vi "Setup.vi"(11 "Event Transport in":refnum<class "Event Transport.lvclass">) -> (0 "Error out":errorcluster, 3 "Event Transport out":refnum<class "Event Transport.lvclass">)   [LabVIEW 2020, in "jettl.lvlib" / "Event Transport.lvlib" / "Event Transport.lvclass"]
uses:
  Event Transport.lvclass
  Msg/Msg.lvclass
  Event Transport.lvclass/Event Transport.ctl
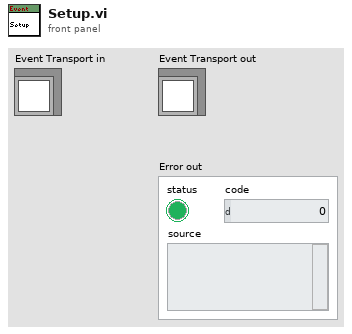
[diagram p1: front panel]
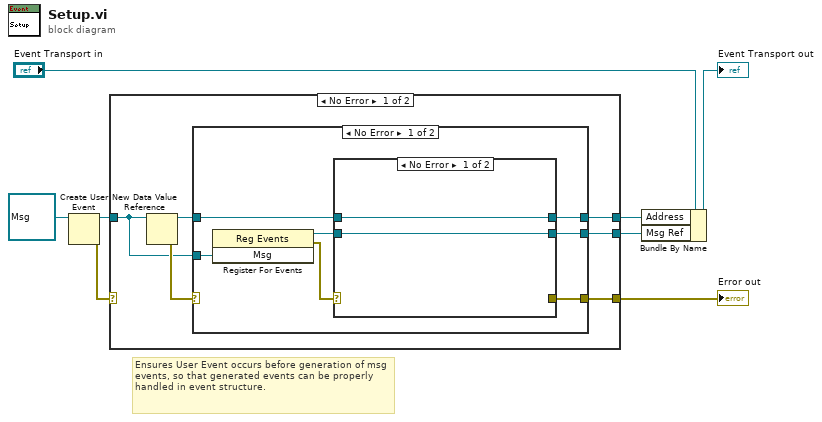
[diagram p0: block diagram]
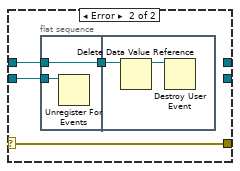
[diagram p2: hidden frame]
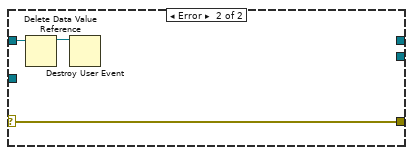
[diagram p3: hidden frame]
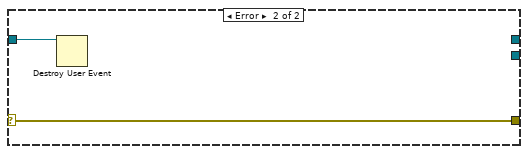
[diagram p4: hidden frame]
diagram:
  # "Ensures User Event occurs before generation of msg events, so that generated events can be properly handled in event structure."
  n1 = Create User Event(user event datatype=refnum<class "Msg.lvclass"> refnum ("Msg")) -> (user event=w5:refnum<user-event>, error out=w4:errorcluster)  [unwired: 1 in]
  n2 = case shown="No Error" w4 {
    selector: w4 -> [_ w36]
    tunnel: [w13 w36] -> w3
    tunnel: w5 -> [w9 w35]
    tunnel: [w11 _] -> w2
    tunnel: [w10 _] -> w1
    frame No Error {
      n3 = New Data Value Reference(data value=w9) -> (data value reference=w12:refnum<data-value>, error out=w14:errorcluster)  [unwired: 1 in]
      n4 = case shown="No Error" w14 {
        selector: w14 -> [_ w34]
        tunnel: [w15 w34] -> w13
        tunnel: w12 -> [w16 w33]
        tunnel: [w17 _] -> w11
        tunnel: [w19 _] -> w10
        tunnel: w9 -> [w18 _]
        frame No Error {
          n5 = register-events(w18) -> (reference out=w20:refnum<event-registration>, error out=w21:errorcluster)  [unwired: 2 in]
          n6 = case shown="No Error" w21 {
            selector: w21 -> [_ w27]
            tunnel: [_ w27] -> w15
            tunnel: [w23 _] -> w19
            tunnel: w20 -> [w23 w26]
            tunnel: [w22 _] -> w17
            tunnel: w16 -> [w22 w24]
            frame No Error {
            }
            frame Error {
              n7 = flat-sequence {
                tunnel: w26 -> [w29]
                tunnel: [w28] -> w25
                tunnel: w24 -> [w28]
                tunnel: w25 -> [w31]
                frame #0 {
                  n8 = Unregister For Events(event registration refnum=w29) -> ()  [unwired: 1 in, 1 out]
                }
                frame #1 {
                  n9 = Delete Data Value Reference(data value reference=w31) -> (data value=w30:refnum<user-event>)  [unwired: 1 in, 1 out]
                  n10 = Destroy User Event(user event=w30) -> ()  [unwired: 1 in, 1 out]
                }
              }
            }
          }
        }
        frame Error {
          n11 = Delete Data Value Reference(data value reference=w33) -> (data value=w32:refnum<user-event>)  [unwired: 1 in, 1 out]
          n12 = Destroy User Event(user event=w32) -> ()  [unwired: 1 in, 1 out]
        }
      }
    }
    frame Error {
      n13 = Destroy User Event(user event=w35) -> ()  [unwired: 1 in, 1 out]
    }
  }
  "Error out" <- w3
  n14 = Bundle By Name(cluster="Event Transport in", "Address"=w2, "Msg Ref"=w1) -> (→"Event Transport out":refnum<class "Event Transport.lvclass">)
